vi "pressure_sensor_model.vi"(10 "input(A)":dbl) -> (2 "output(bar)":dbl)   [LabVIEW 2020]
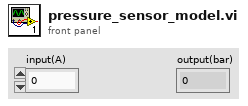
[diagram p1: front panel]
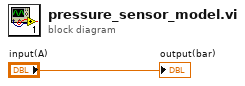
[diagram p0: block diagram]
diagram:
  "output(bar)" <- "input(A)"
